vi "Populate_Do.vi"(8 "error in (no error)":errorcluster, 9 "Value":string, 10 "Lower case name":string, 11 "PPL Class Test in":refnum<class "PPL Class Test.lvclass">) -> (0 "error out":errorcluster, 1 "Success?":bool, 3 "PPL Class Test out":refnum<class "PPL Class Test.lvclass">)   [LabVIEW 2020, in "ProjectBuilder.lvlib" / "PPL Class Test.lvclass"]
doc: "Override to populate private data from strings.\n\nThe default implementation does nothing but return 'Success?'=True."
uses:
  PPL Class Test.lvclass
  ProjectBuilder.lvlib
  PPL/HDH.ClassLoader.lvlibp
  PPL Class Test Plugin/PPL Class Test Plugin.lvclass
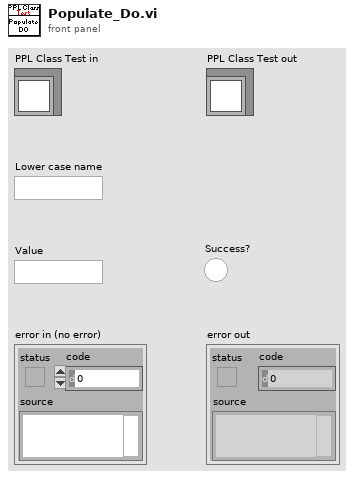
[diagram p1: front panel]
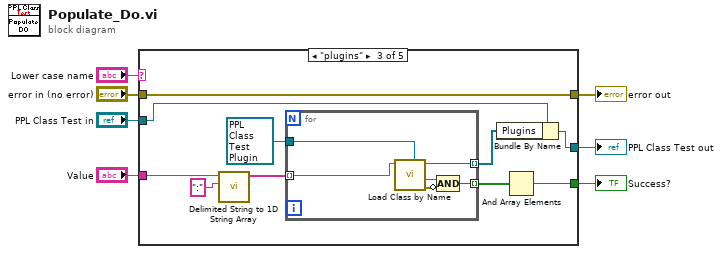
[diagram p0: block diagram]
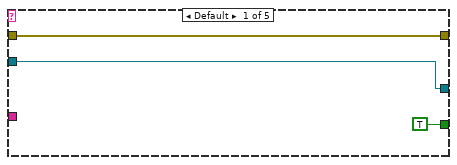
[diagram p2: hidden frame]
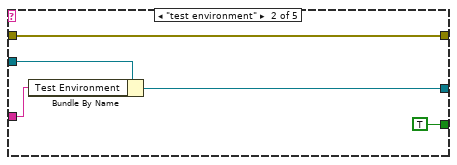
[diagram p3: hidden frame]
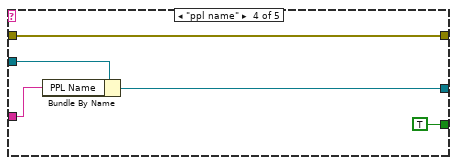
[diagram p4: hidden frame]
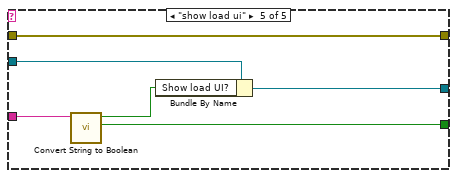
[diagram p5: hidden frame]
diagram:
  n1 = case shown="\"plugins\"" "Lower case name" {
    tunnel: [TRUE TRUE w19 TRUE w39] -> w6
    tunnel: [w9 w11 w25 w32 w40] -> w5
    tunnel: "error in (no error)" -> [w9 w11 w25 w32 w40]
    tunnel: [w8 w14 w23 w35 w41] -> w3
    tunnel: "PPL Class Test in" -> [w8 w15 w24 w36 w42]
    tunnel: "Value" -> [_ w13 w22 w34 w38]
    frame Default {
    }
    frame "test environment" {
      n2 = Bundle By Name(cluster=w15, "Test Environment"=w13) -> (w14:refnum<class "PPL Class Test.lvclass">)
    }
    frame "plugins" {
      n3 = call <vilib>:"Delimited String to 1D String Array.vi"("delimiter"=":", "delimited string"=w22) -> ("string array"=w18:string[])  [unwired: 9 in]
      n4 = for {
        tunnel: w18 -> [w31] mode=indexing
        tunnel: [w28] -> w20 mode=indexing
        tunnel: refnum<class "PPL Class Test Plugin.lvclass"> refnum ("ProjectBuilder.lvlib:PPL Class Test Plugin.lvclass") -> [w27]
        tunnel: [w26] -> w16 mode=indexing
        n5 = call "Load Class by Name.vi"("Class Type"=w27, "Base Class Name"=w31) -> ("error out"=w29:errorcluster, "Load and Type Success?"=w30:bool, "Loaded Class"=w26:refnum<class "PPL Class Test Plugin.lvclass">)  [unwired: 6 in, 1 out]
        n6 = Compound Arithmetic op=AND(w30, invert w29) -> (w28:bool)
      }
      n7 = Bundle By Name(cluster=w24, "Plugins"=w16) -> (w23:refnum<class "PPL Class Test.lvclass">)
      n8 = And Array Elements(Boolean array=w20) -> (logical AND=w19:bool)
    }
    frame "ppl name" {
      n9 = Bundle By Name(cluster=w36, "PPL Name"=w34) -> (w35:refnum<class "PPL Class Test.lvclass">)
    }
    frame "show load ui" {
      n10 = call "Convert String to Boolean.vi"("String"=w38) -> ("Valid string?"=w39:bool, "Boolean value"=w37:bool)  [unwired: 9 in]
      n11 = Bundle By Name(cluster=w42, "Show load UI?"=w37) -> (w41:refnum<class "PPL Class Test.lvclass">)
    }
  }
  "error out" <- w5
  "PPL Class Test out" <- w3
  "Success?" <- w6
